vi "WireUpReadVI.vi"(8 "error in (no error)":errorcluster, 10 "New Control Ref":refnum<vi>, 11 "BaseAccessorScripter in":refnum<class "BaseAccessorScripter.lvclass">) -> (0 "error out":errorcluster, 2 "Multiframe Stuct out":refnum<vi>, 3 "BaseAccessorScripter out":refnum<class "BaseAccessorScripter.lvclass">)   [LabVIEW 2021, in "MemberVICreation.lvlib" / "BaseAccessorScripter.lvclass"]
uses:
  <resource>/Framework/Providers/LVClassLibrary/NewAccessors/BaseAccessorScripter/BaseAccessorScripter.lvclass
  <resource>/Framework/Providers/LVClassLibrary/NewAccessors/BaseAccessorScripter/BaseAccessorScripter.lvclass/BaseAccessorScripter.ctl
  <resource>/Framework/Providers/LVClassLibrary/NewAccessors/MemberVICreation.lvlib
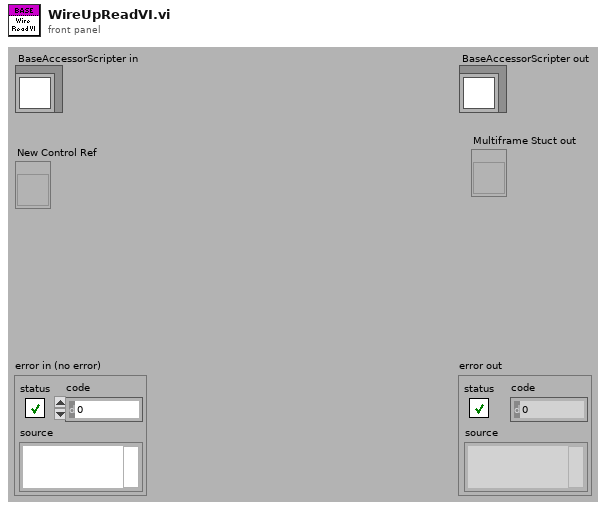
[diagram p1: front panel]
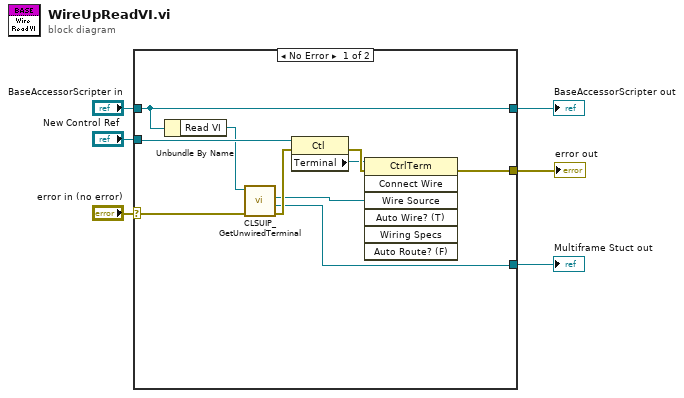
[diagram p0: block diagram]
diagram:
  n1 = case shown="No Error" "error in (no error)" {
    selector: "error in (no error)" -> [w11 w18]
    tunnel: [w8 w18] -> w5
    tunnel: [w13 w17] -> w3
    tunnel: "BaseAccessorScripter in" -> [w13 w17]
    tunnel: "New Control Ref" -> [w16 _]
    tunnel: [w7 _] -> w1
    frame No Error {
      n2 = Unbundle By Name(w13) -> ("Read VI"=w12:refnum<vi>)
      n3 = call <resource>:"CLSUIP_GetUnwiredTerminal.vi"("error in (no error)"=w11, "VI Refnum"=w12) -> ("error out"=w10:errorcluster, "Multiframe Stuct out"=w7:refnum<vi>, "Outer Terminal Ref"=w9:refnum<vi>)  [unwired: 7 out]
      n4 = property class="Ctl"(reference=w16, error in=w10) -> (error out=w15:errorcluster, "Terminal"=w14:refnum<vi>)  [unwired: 1 out]
      n5 = invoke class="CtrlTerm" method="Connect Wire"(reference=w14, error in=w15, "Wire Source"=w9) -> (error out=w8:errorcluster)  [unwired: 4 in, 6 out]
    }
    frame Error {
    }
  }
  "error out" <- w5
  "BaseAccessorScripter out" <- w3
  "Multiframe Stuct out" <- w1
